vi "Namen cRio Daten.vi"(4 "Password":string="iag", 6 "User Name":string="iag", 7 "IP Adresse":string, 8 "error in":errorcluster, 11 "startup":bool) -> (0 "error out":errorcluster, 2 "Pfad cRio":string, 3 "Dateien FTP":string[](array[string]))   [LabVIEW 2020, in "FTP WebDAV.lvlib"]
uses:
  FTP WebDAV.lvlib
  Aktionen FTP WebDAV.ctl
  <vilib>/FTP/NI_FTP.lvlib
  <vilib>/WebDAVClient/NI_WebDAV.lvlib
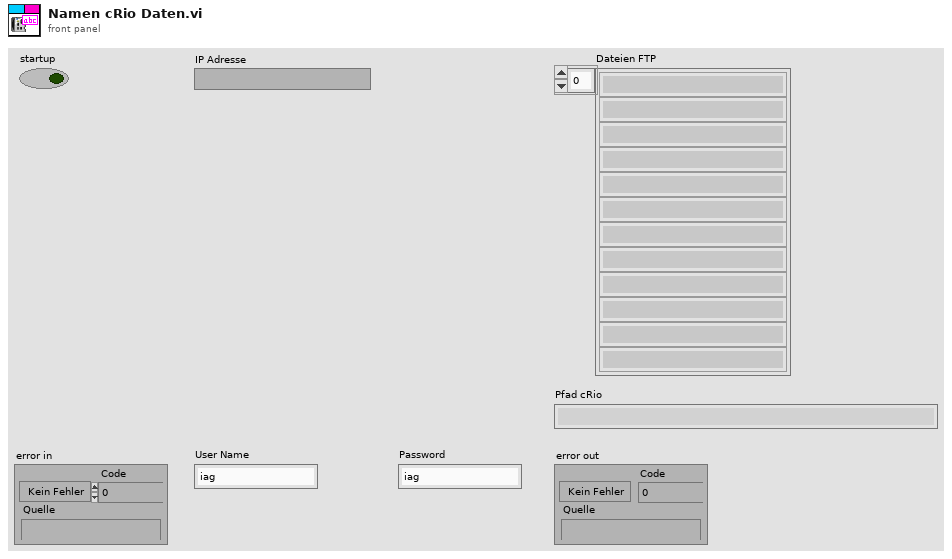
[diagram p1: front panel]
types:
  T1 = typedef "FTP WebDAV.lvlib/Aktionen FTP WebDAV.ctl" = enum16{"lesen", "erkennen"}
  T2 = typedef "FTP WebDAV.lvlib/Enum FTP WebDAV.ctl" = enum16{" nix", "ftp", "webDAV"}
  T3 = typedef "NI_WebDAV.lvlib/SessionHandle.ctl" = refnum<k1>
  T4 = typedef "NI_WebDAV.lvlib/FileInfo.ctl" = cluster{"type":string, "size":u64, "last modification":timestamp, "display name":string, "uri":string}
  T5 = typedef "NI_FTP.lvlib/FTP Session.ctl" = refnum<k5>
  T6 = typedef "NI_FTP.lvlib/FTP File Info.ctl" = cluster{"type":enum16{"unknown", "file", "dir", "link"}, "permissions":string, "owner":string, "group":string, "size":i32, "date":string, "name":string, "link name":string}
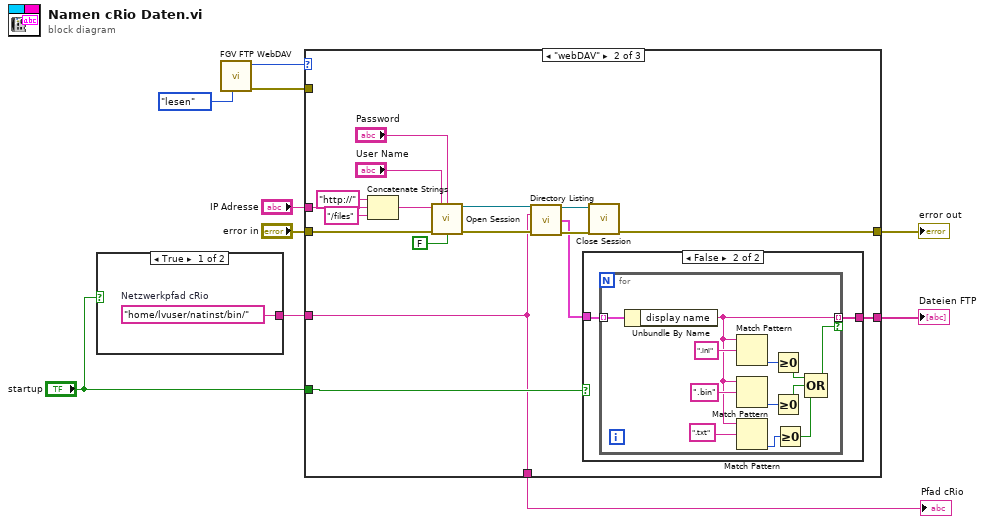
[diagram p0: block diagram]
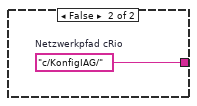
[diagram p2: hidden frame]
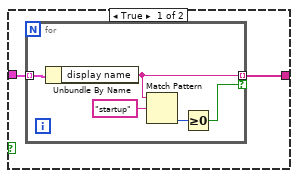
[diagram p4: hidden frame]
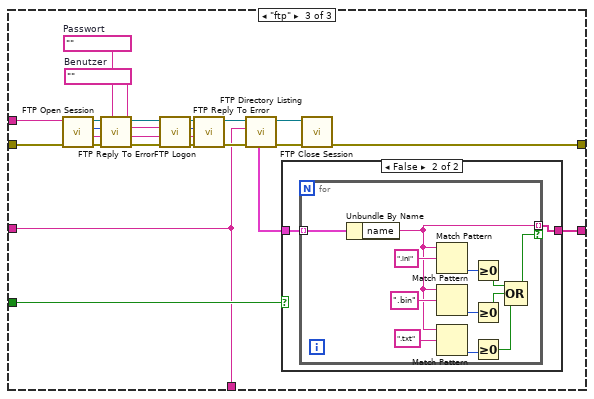
[diagram p5: hidden frame]
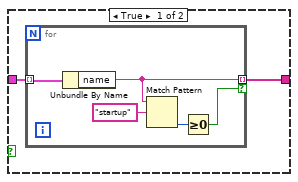
[diagram p6: hidden frame]
diagram:
  n1 = case shown="True" "startup" {
    tunnel: [w11 w12] -> w1
    frame True {
      w11 = "home/lvuser/natinst/bin/"  # Netzwerkpfad cRio
    }
    frame False {
      w12 = "c/KonfigIAG/"  # Netzwerkpfad cRio
    }
  }
  n2 = call "FGV FTP WebDAV.vi"("Aktionen"=Aktionen_FTP_WebDAV."lesen") -> ("Fehler (Ausgang)"=w3:errorcluster, "ftp webDAV"=w5:T2)  [unwired: 6 in, 3 out]
  n3 = case shown="\"webDAV\"" w5 {
    tunnel: [_ w14 w52] -> w10
    tunnel: "error in" -> [_ w30 w74]
    tunnel: [w13 w29 w73] -> w8
    tunnel: "IP Adresse" -> [_ w28 w72]
    tunnel: "startup" -> [_ w17 w53]
    tunnel: [_ w18 w54] -> w4
    tunnel: w3 -> [w13 _ _]
    tunnel: w1 -> [_ w14 w52]
    frame " nix", Default {
    }
    frame "webDAV" {
      n4 = Concatenate Strings("http://" ("String"), w28, "/files" ("String")) -> (w24:string)
      n5 = call <vilib>:"Open Session.vi"("host uri prefix"=w24, "username"="User Name", "password"="Password", "error in (no error)"=w30, "verify server?"=FALSE) -> ("session handle out"=w26:T3, "error out"=w27:errorcluster)  [unwired: 9 in]
      n6 = call <vilib>:"Directory Listing.vi"("session handle"=w26, "relative uri"=w14, "error in (no error)"=w27) -> ("session handle out"=w21:T3, "file list"=w19:T4[], "error out"=w20:errorcluster)  [unwired: 9 in, 1 out]
      n7 = case shown="False" w17 {
        tunnel: w19 -> [w32 w39]
        tunnel: [w31 w38] -> w18
        frame True {
          n8 = for {
            tunnel: w32 -> [w37] mode=indexing
            tunnel: [w36] -> w31 mode=indexing if=w34
            n9 = Unbundle By Name(w37) -> ("display name"=w36:string)
            n10 = Match Pattern(string=w36, regular expression="startup" ("Regulärer Ausdruck")) -> (offset past match=w35:i32)  [unwired: 1 in, 3 out]
            n11 = Greater Or Equal To 0?(x=w35) -> (x >= 0?=w34:bool)
          }
        }
        frame False {
          n12 = for {
            tunnel: w39 -> [w51] mode=indexing
            tunnel: [w43] -> w38 mode=indexing if=w44
            n13 = Unbundle By Name(w51) -> ("display name"=w43:string)
            n14 = Match Pattern(string=w43, regular expression=".ini" ("Regulärer Ausdruck")) -> (offset past match=w50:i32)  [unwired: 1 in, 3 out]
            n15 = Match Pattern(string=w43, regular expression=".bin" ("Regulärer Ausdruck")) -> (offset past match=w48:i32)  [unwired: 1 in, 3 out]
            n16 = Match Pattern(string=w43, regular expression=".txt" ("Regulärer Ausdruck")) -> (offset past match=w41:i32)  [unwired: 1 in, 3 out]
            n17 = Greater Or Equal To 0?(x=w50) -> (x >= 0?=w45:bool)
            n18 = Greater Or Equal To 0?(x=w48) -> (x >= 0?=w46:bool)
            n19 = Greater Or Equal To 0?(x=w41) -> (x >= 0?=w40:bool)
            n20 = Compound Arithmetic op=OR ("Mehrfacharithmetik")(w45, w46, w40) -> (w44:bool)
          }
        }
      }
      n21 = call <vilib>:"Close Session.vi"("session handle"=w21, "error in (no error)"=w20) -> ("error out"=w29:errorcluster)  [unwired: 13 in]
    }
    frame "ftp" {
      w57 = ""  # Passwort
      w56 = ""  # Benutzer
      n22 = call <vilib>:"FTP Open Session.vi"("error in (no error)"=w74, "address"=w72) -> ("error out"=w62:errorcluster, "reply string"=w61:string, "reply code"=w60:i32, "ftp session"=w59:T5)  [unwired: 6 in]
      n23 = call <vilib>:"FTP Reply To Error.vi"("error in (no error)"=w62, "reply string in"=w61, "reply code in"=w60, "ftp session"=w59) -> ("error out"=w63:errorcluster, "ftp session out"=w58:T5)  [unwired: 2 out]
      n24 = call <vilib>:"FTP Logon.vi"("error in (no error)"=w63, "password"=w57, "user"=w56, "ftp session"=w58) -> ("error out"=w67:errorcluster, "reply string"=w66:string, "reply code"=w65:i32, "ftp session out"=w64:T5)  [unwired: 4 in]
      n25 = call <vilib>:"FTP Reply To Error.vi"("error in (no error)"=w67, "reply string in"=w66, "reply code in"=w65, "ftp session"=w64) -> ("error out"=w68:errorcluster, "ftp session out"=w69:T5)  [unwired: 2 out]
      n26 = call <vilib>:"FTP Directory Listing.vi"("error in (no error)"=w68, "directory path"=w52, "ftp session"=w69) -> ("error out"=w70:errorcluster, "ftp session out"=w71:T5, "dir list"=w55:T6[])  [unwired: 4 in, 2 out]
      n27 = case shown="False" w53 {
        tunnel: w55 -> [w76 w83]
        tunnel: [w75 w82] -> w54
        frame True {
          n28 = for {
            tunnel: w76 -> [w81] mode=indexing
            tunnel: [w80] -> w75 mode=indexing if=w78
            n29 = Unbundle By Name(w81) -> ("name"=w80:string)
            n30 = Match Pattern(string=w80, regular expression="startup" ("Regulärer Ausdruck")) -> (offset past match=w79:i32)  [unwired: 1 in, 3 out]
            n31 = Greater Or Equal To 0?(x=w79) -> (x >= 0?=w78:bool)
          }
        }
        frame False {
          n32 = for {
            tunnel: w83 -> [w95] mode=indexing
            tunnel: [w87] -> w82 mode=indexing if=w88
            n33 = Unbundle By Name(w95) -> ("name"=w87:string)
            n34 = Match Pattern(string=w87, regular expression=".ini" ("Regulärer Ausdruck")) -> (offset past match=w94:i32)  [unwired: 1 in, 3 out]
            n35 = Match Pattern(string=w87, regular expression=".bin" ("Regulärer Ausdruck")) -> (offset past match=w92:i32)  [unwired: 1 in, 3 out]
            n36 = Match Pattern(string=w87, regular expression=".txt" ("Regulärer Ausdruck")) -> (offset past match=w85:i32)  [unwired: 1 in, 3 out]
            n37 = Greater Or Equal To 0?(x=w94) -> (x >= 0?=w89:bool)
            n38 = Greater Or Equal To 0?(x=w92) -> (x >= 0?=w90:bool)
            n39 = Greater Or Equal To 0?(x=w85) -> (x >= 0?=w84:bool)
            n40 = Compound Arithmetic op=OR ("Mehrfacharithmetik")(w89, w90, w84) -> (w88:bool)
          }
        }
      }
      n41 = call <vilib>:"FTP Close Session.vi"("error in (no error)"=w70, "ftp session"=w71) -> ("error out"=w73:errorcluster)  [unwired: 6 in, 3 out]
    }
  }
  "error out" <- w8
  "Dateien FTP" <- w4
  "Pfad cRio" <- w10
